vi "Oblicz zakres SVG.vi"(4 "napiecie progu Low (0,1V)":dbl=0.1 format="%#_13g", 6 "napiecie progu High (1,9V)":dbl=1.9 format="%#_13g", 7 "Akcja":T1, 8 "error in (no error)":errorcluster, 11 "Kanaly nieprzetw in":T2) -> (0 "error out":errorcluster, 2 "Przekroczone Low":bool[](array[boolean]), 3 "Przekroczone High":bool[](array[boolean]))   [LabVIEW 2013]
doc: "Use this template to build a VI to use as a subVI."
uses:
  Kontrolki/Przetwarzanie/Kanaly.ctl
  Kontrolki/FVGs/FVG akcje podstawowa.ctl
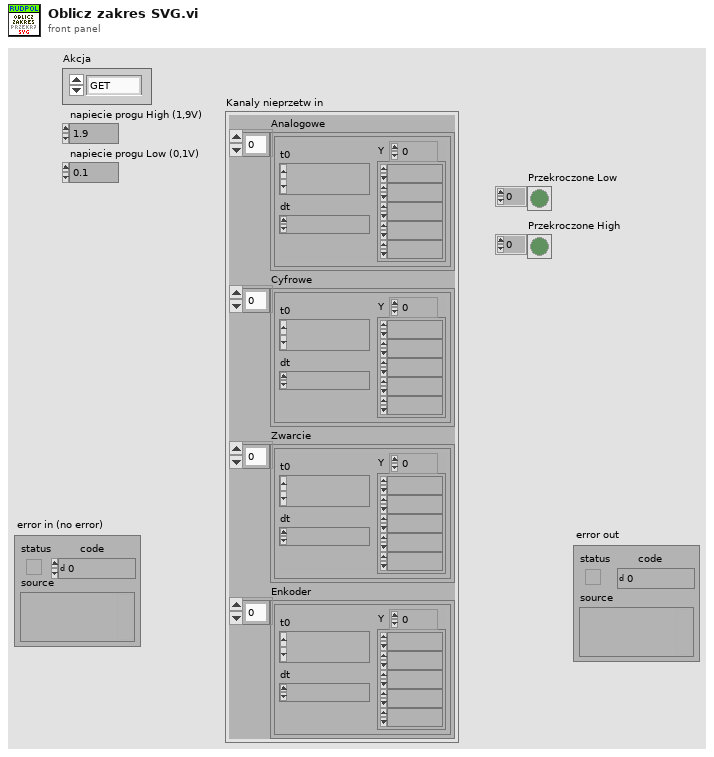
[diagram p1: front panel]
types:
  T1 = typedef "FVG akcje podstawowa.ctl" = enum16{"GET", "SET"}
  T2 = typedef "Kanaly.ctl" = cluster{"Analogowe":waveform(dbl)[], "Cyfrowe":waveform(dbl)[], "Zwarcie":waveform(dbl)[], "Enkoder":waveform(dbl)[]}
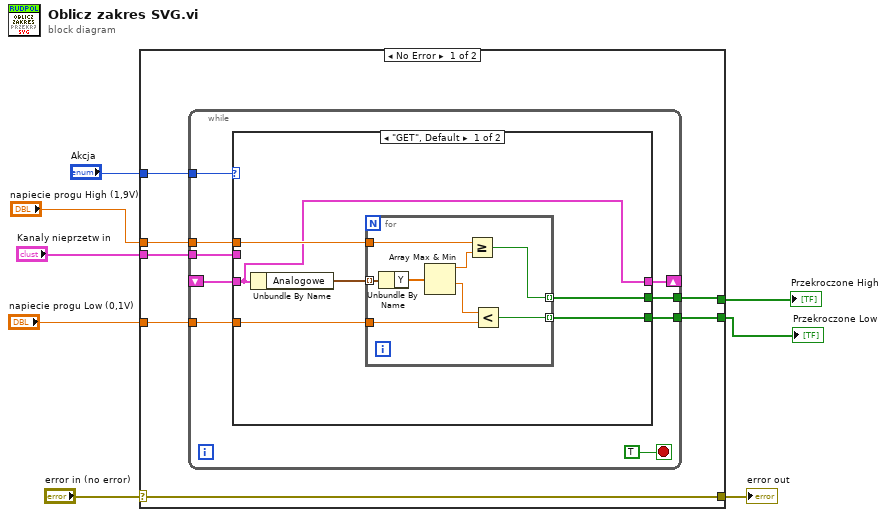
[diagram p0: block diagram]
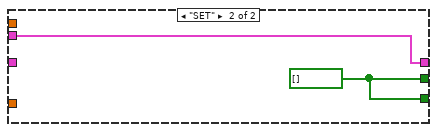
[diagram p2: hidden frame]
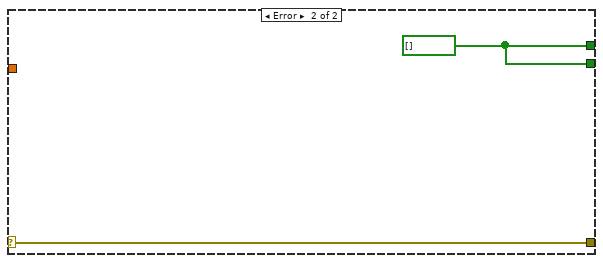
[diagram p3: hidden frame]
diagram:
  n1 = case shown="No Error" "error in (no error)" {
    selector: "error in (no error)" -> [w15 w42]
    tunnel: [w15 w42] -> w7
    tunnel: "Kanaly nieprzetw in" -> [w14 _]
    tunnel: "Akcja" -> [w13 _]
    tunnel: "napiecie progu High (1,9V)" -> [w12 _]
    tunnel: "napiecie progu Low (0,1V)" -> [w11 _]
    tunnel: [w10 w41] -> w2
    tunnel: [w9 w41] -> w1
    frame No Error {
      n2 = while {
        tunnel: w14 -> [w21]
        tunnel: w13 -> [w23]
        shift-right: [w22] -> _
        shift-left: _ -> [w20]
        tunnel: w12 -> [w19]
        tunnel: w11 -> [w18]
        tunnel: [w17] -> w10
        tunnel: [w16] -> w9
        stop <- TRUE stop-if-true
        n3 = case shown="\"GET\", Default" w23 {
          tunnel: [w28 w40] -> w22
          tunnel: w21 -> [_ w40]
          tunnel: w20 -> [w28 _]
          tunnel: w19 -> [w29 _]
          tunnel: w18 -> [w27 _]
          tunnel: [w26 w39] -> w17
          tunnel: [w25 w39] -> w16
          frame "GET", Default {
            n4 = Unbundle By Name(w28) -> ("Analogowe"=w30:waveform(dbl)[])
            n5 = for {
              tunnel: w30 -> [w38] mode=indexing
              tunnel: w29 -> [w32]
              tunnel: w27 -> [w35]
              tunnel: [w31] -> w26 mode=indexing
              tunnel: [w34] -> w25 mode=indexing
              n6 = Unbundle By Name(w38) -> ("Y"=w37:dbl[])
              n7 = Array Max & Min(array=w37) -> (max value=w33:dbl, min value=w36:dbl)  [unwired: 2 out]
              n8 = Greater Or Equal?(x=w32, y=w33) -> (x >= y?=w31:bool)
              n9 = Less?(x=w36, y=w35) -> (x < y?=w34:bool)
            }
          }
          frame "SET" {
            w39 = bool[] []
          }
        }
      }
    }
    frame Error {
      w41 = bool[] []
    }
  }
  "error out" <- w7
  "Przekroczone High" <- w2
  "Przekroczone Low" <- w1
